vi "LearningVI.vi"() -> ()   [LabVIEW 2013]
panel:
  out "P2P t-Avg":dbl
  out "Peak-to-Peak":dbl
  out "DC NoAvg":dbl
  out "DC t-Avg":dbl
  out "Waveform Chart":dynamicdata(graph)
  in  "stop (F)":bool
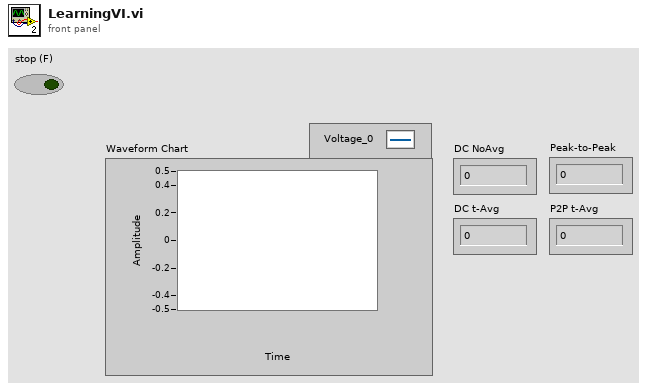
[diagram p1: front panel]
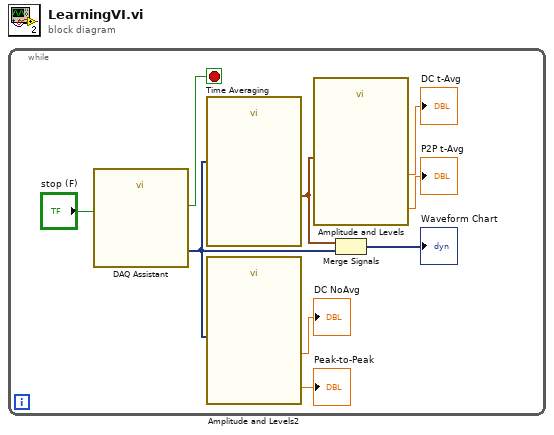
[diagram p0: block diagram]
diagram:
  n1 = while {
    stop <- w8 stop-if-true
    n2 = call "DAQ Assistant"("stop (F)"="stop (F)") -> ("data"=w3:dynamicdata, "stopped"=w8:bool)  [unwired: 15 in, 2 out]
    n3 = call "Time Averaging"("input signal"=w3) -> ("time avg. signal"=w7:waveform(dbl))  [unwired: 15 in, 3 out]
    n4 = call "Amplitude and Levels2"("input signal"=w3) -> ("dc"=→"DC NoAvg":dbl, "peak-peak"=→"Peak-to-Peak":dbl)  [unwired: 15 in, 2 out]
    n5 = call "Amplitude and Levels"("input signal"=w7) -> ("dc"=→"DC t-Avg":dbl, "peak-peak"=→"P2P t-Avg":dbl)  [unwired: 15 in, 2 out]
    n6 = Merge Signals(w7, w3) -> (→"Waveform Chart":dynamicdata)
  }
